vi "VolatusAPI.vi"(11 "Module in":refnum<class "Module.lvclass">) -> (2 "VolatusAPI":refnum<class "VolatusAPI.lvclass">, 3 "Module out":refnum<class "Module.lvclass">)   [LabVIEW 2020, in "Volatus.lvlib" / "Module.lvclass"]
uses:
  Module.lvclass
  Module.lvclass/Module.ctl
  VolatusAPI/VolatusAPI.lvclass
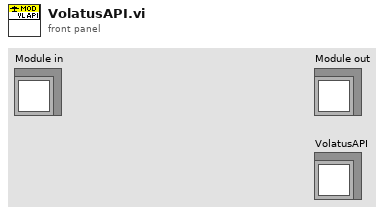
[diagram p1: front panel]
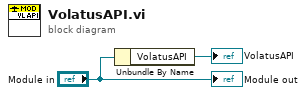
[diagram p0: block diagram]
diagram:
  n1 = Unbundle By Name("Module in") -> ("VolatusAPI"=→"VolatusAPI":refnum<class "VolatusAPI.lvclass">)
  "Module out" <- "Module in"
